vi "ziExample-Scope.vi"() -> ()   [LabVIEW 2009]
doc: "Control a Zurich instrument device via the LabOne Labview API. \nRequirements: Zurich Instruments MFLI, HF2 or UHFLI \nThis example retrieves scope data from a Zurich Instruments instrument.\n\n© Zurich Instruments AG, www.zhinst.com"
uses:
  <instrlib>/Zurich Instruments LabOne/Public/Configure/ziSetValueDouble.vi
  <instrlib>/Zurich Instruments LabOne/Public/Configure/ziGetValueString.vi
  <instrlib>/Zurich Instruments LabOne/Public/Configure/ziSetValueDoubleArray.vi
  <instrlib>/Zurich Instruments LabOne/Public/Configure/ziGetValueDouble.vi
  <instrlib>/Zurich Instruments LabOne/Public/Data/ziGetEventScopeWaveEX.vi
  <instrlib>/Zurich Instruments LabOne/Zurich Instruments LabOne.lvlib
  <vilib>/Analysis/NI_AALPro.lvlib
panel:
  out "ScopeWave Out":T1(array[cluster])
  out "Error Out":errorcluster
  in  "Address":string="DEV"
  out "FFT":T2(graph)
  out "Selected Device":string
  out "Waveform":cluster{"dt (?)":dbl, "dt (s)":dbl, dbl[]}[](graph)
  in  "stop":bool
  # "ziExample-Scope.vi:\nThis example is legacy and please use ziExample-Module-Scope.vi"
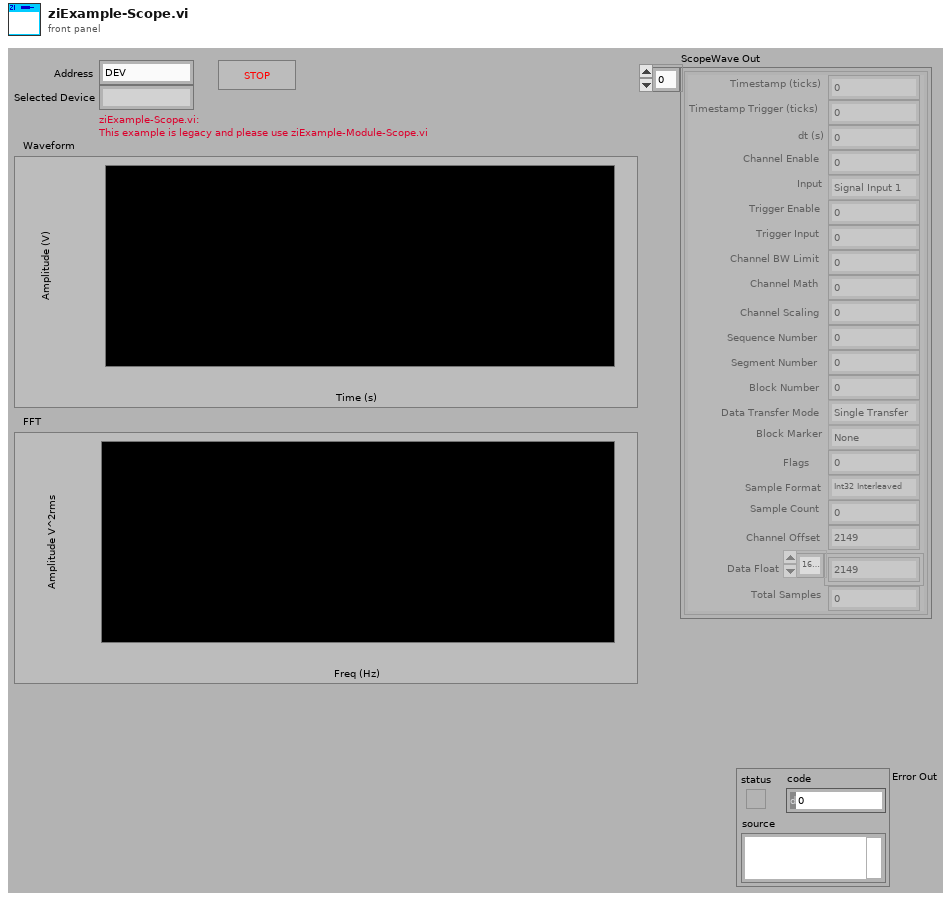
[diagram p1: front panel]
types:
  T1 = cluster{"Timestamp (ticks)":u64, "Timestamp Trigger (ticks)":u64, "dt (s)":dbl, "Channel Enable":u8, "Input":enum8{"Signal Input 1", "Signal Input 2", "Trigger Input 1", "Trigger Input 2", "Aux Output 1", "Aux Output 2", "Aux Output 3", "Aux Output 4", "Aux Input 1", "Aux Input 2"}, "Trigger Enable":u64, "Trigger Input":u64, "Channel BW Limit":u8, "Channel Math":u8, "Channel Scaling":sgl, "Sequence Number":u32, "Segment Number":u32, "Block Number":u32, "Data Transfer Mode":enum8{"Single Transfer", "Block Transfer", "Continuous Transfer", "FFT Single Transfer"}, "Block Marker":enum8{"None", "End of Block"}, "Flags":u8, "Sample Format":enum8{"Int16", "Int32", "Float32", "reserved", "Int16 Interleaved", "Int32 Interleaved", "Float32 Interleaved"}, "Sample Count":u32, "Channel Offset":dbl, "Data Float":sgl[], "Total Samples":u64}[]
  T2 = cluster{"dt (?)":dbl, "df":dbl, "Power Spectrum (V^2 rms)":dbl[]}[]
  T3 = typedef "Zurich Instruments LabOne.lvlib/ziTypeHandle.ctl" = cluster{"handleValid":bool, "Conn":u64, "Path Prefix":string, "Handle":u64, "Connected":bool, "Clockbase(s)":dbl}
  T4 = typedef "Zurich Instruments LabOne.lvlib/ziTypePollType.ctl" = enum16{"NONE", "DOUBLE_DATA", "INTEGER_DATA", "DEMOD_SAMPLE", "SCOPE_WAVE_HF2", "AUXIN_SAMPLE", "DIO_SAMPLE", "BYTE_ARRAY", "PWA_WAVE", "9", "10", "11", "12", "13", "14", "15", "TREE_CHANGE_DEPRI", "17", "ERROR", "19", "20", "21", "22", "23", "24", "25", "26", "27", "28", "29", "30", "31", "DOUBLE_DATA_TS", "INTEGER_DATA_TS", "34", "SCOPE_WAVE", "SCOPE_WAVE_EX", "37", "BYTE_ARRAY_TS", "39", "40", "41", "42", "43", "44", "45", "CNT_DATA", "47", "TREE_CHANGE", "49", "50", "51", "52", "53", "54", "55", "56", "57", "58", "59", "60", "61", "62", "63", "SWEEPER_DATA", "SPECTRUM_DATA", "ADVISOR_DATA", "VECTOR_DATA", "IMP_DATA"}
  T5 = cluster{"dt (?)":dbl, "df":dbl, "Power Spectrum (V^2 rms)":dbl[]}
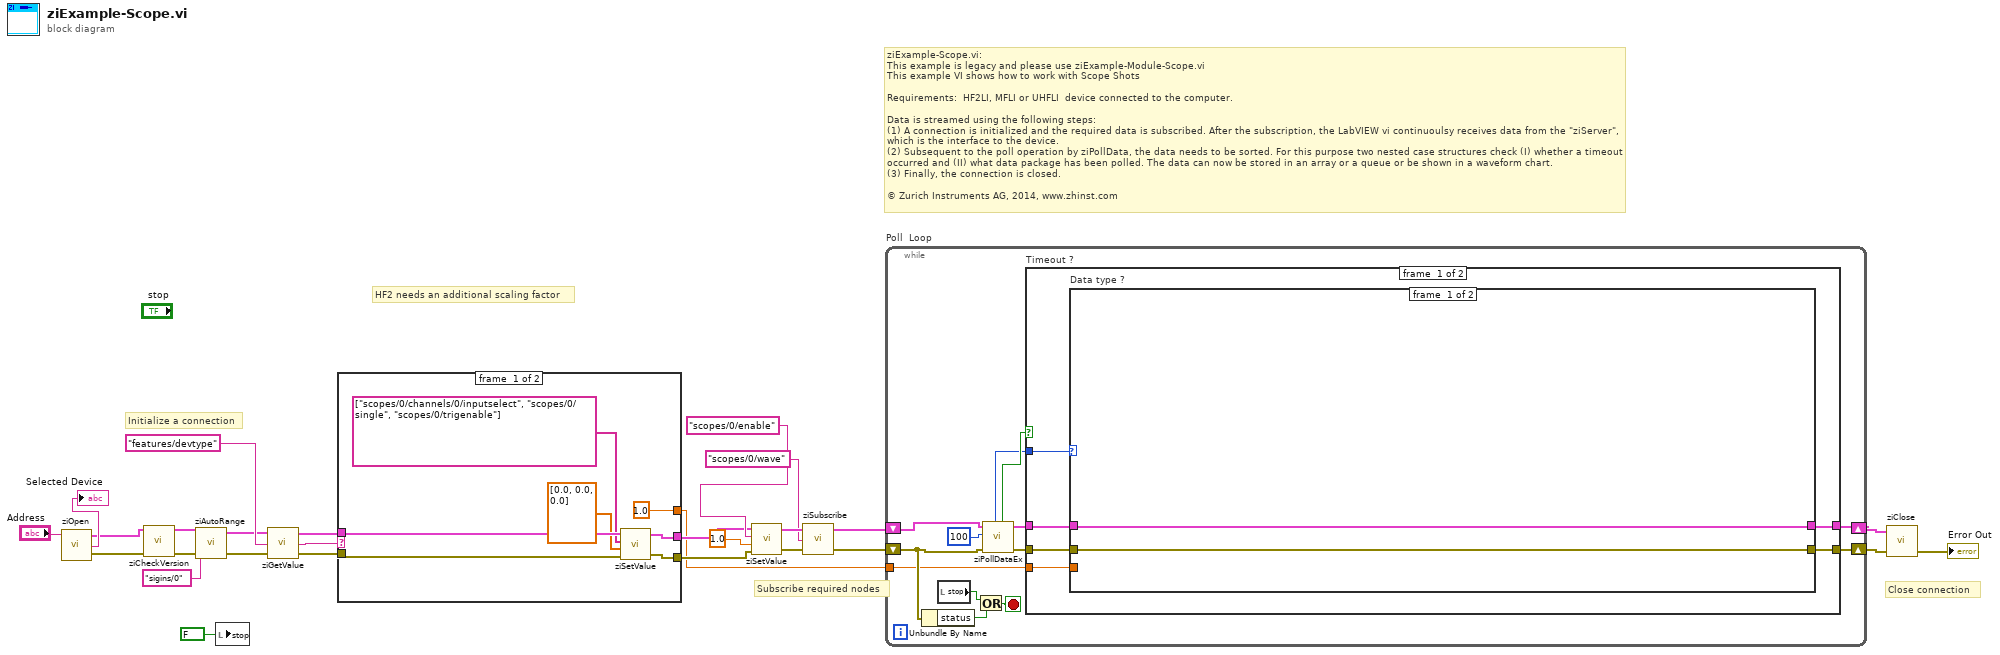
[diagram p0: block diagram]
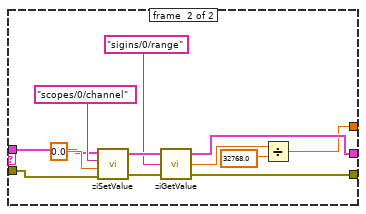
[diagram p2: hidden frame]
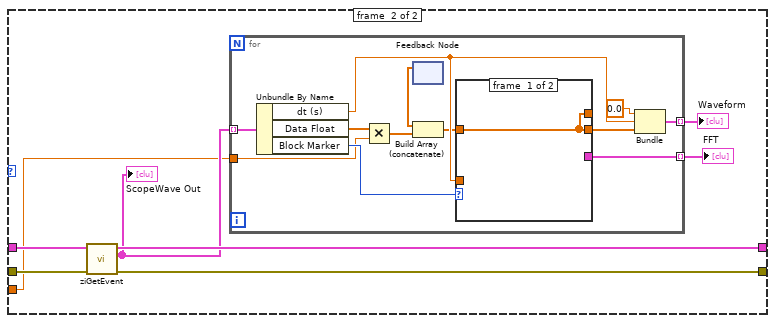
[diagram p3: hidden frame]
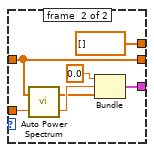
[diagram p4: hidden frame]
diagram:
  # "Close connection"
  # "HF2 needs an additional scaling factor"
  # "Initialize a connection"
  # "Subscribe required nodes"
  # "ziExample-Scope.vi:\nThis example is legacy and please use ziExample-Module-Scope.vi\nThis example VI shows how to work with Scope Shots\n\nRequirements:  HF2LI, MFLI or UHFLI  device connected to the computer.\n\nData is streamed using the following steps:\n(1) A connection is initialized and the required data is subscribed. After the subscription, the LabVIEW vi continuoulsy receives data from the \"ziServer\", which is the interface to the device. \n(2) Subsequent to the poll operation by ziPollData, the data needs to be sorted. For this purpose two nested case structures check (I) whether a timeout occurred and (II) what data package has been polled. The data can now be stored in an array or a queue or be shown in a waveform chart. \n(3) Finally, the connection is closed. \n\n© Zurich Instruments AG, 2014, www.zhinst.com"
  n1 = call <instrlib>:"ziOpen.vi"("Address"="Address") -> ("Error Out"=w2:errorcluster, "Selected Device"=→"Selected Device":string, "HandleOut"=w1:T3)  [unwired: 1 in, 2 out]
  n2 = call <instrlib>:"ziCheckVersion.vi"("Handle In"=w1, "Error In"=w2) -> ("Handle Out"=w4:T3, "Error Out"=w3:errorcluster)  [unwired: 11 in, 1 out]
  n3 = call <instrlib>:"ziAutoRange.vi"("Error in"=w3, "Path"="sigins/0", "Handle in"=w4) -> ("Error out"=w6:errorcluster, "Handle out"=w7:T3)  [unwired: 6 in, 1 out]
  n4 = local write "stop"(FALSE ("Record")) -> ()
  n5 = call-poly <instrlib>:"ziGetValue.vi"("error in"=w6, "Path"="features/devtype", "Handle In"=w7) -> ("error out"=w14:errorcluster, "Value"=w12:string, "Handle Out"=w13:T3)
  n6 = case shown="Default" w12 {
    tunnel: w13 -> [w34 w44]
    tunnel: w14 -> [w33 w43]
    tunnel: [w32 w40] -> w16
    tunnel: [w31 w41] -> w15
    tunnel: [1.0 w36] -> w10
    frame #0 {
      n7 = call-poly <instrlib>:"ziSetValue.vi"("Error In"=w33, "Values"=dbl[] [0.0, 0.0, 0.0], "Paths"=string[] ["scopes/0/channels/0/inputselect", "scopes/0/single", "scopes/0/trigenable"], "Handle In"=w34) -> ("Error Out"=w32:errorcluster, "Handle Out"=w31:T3)  [unwired: 1 in]
    }
    frame #1 {
      n8 = call-poly <instrlib>:"ziSetValue.vi"("Error In"=w43, "Value"=0.0, "Path"="scopes/0/channel", "Handle In"=w44) -> ("Error Out"=w39:errorcluster, "Handle Out"=w42:T3)  [unwired: 1 in]
      n9 = call-poly <instrlib>:"ziGetValue.vi"("error in"=w39, "Path"="sigins/0/range", "Handle in"=w42) -> ("error out"=w40:errorcluster, "Value"=w37:dbl, "Handle out"=w41:T3)
      n10 = Divide(x=w37, y=32768.0) -> (x/y=w36:dbl)
    }
  }
  n11 = call-poly <instrlib>:"ziSetValue.vi"("Error In"=w16, "Value"=1.0, "Path"="scopes/0/enable", "Handle In"=w15) -> ("Error Out"=w20:errorcluster, "Handle Out"=w21:T3)  [unwired: 1 in]
  n12 = call <instrlib>:"ziSubscribe.vi"("error in"=w20, "Path ()"="scopes/0/wave" ("path"), "Handle In"=w21) -> ("error out"=w24:errorcluster, "Handle Out"=w8:T3)  [unwired: 1 in]
  n13 = while "Poll  Loop" {
    shift-right: [w55] -> w25
    shift-left: w8 -> [w59]
    shift-right: [w53] -> w26
    shift-left: w24 -> [w52]
    tunnel: w10 -> [w48]
    stop <- w49 stop-if-true
    n14 = Unbundle By Name(w52) -> ("status"=w51:bool)
    n15 = local read "stop"() -> (w50:bool)
    n16 = Or(x=w50, y=w51) -> (x .or. y?=w49:bool)
    n17 = call <instrlib>:"ziPollDataEx.vi"("error in"=w52, "Timeout ms (50)"=100 ("TimeOut ms (50)"), "Handle In"=w59) -> ("error out"=w54:errorcluster, "Handle Out"=w56:T3, "Timed Out"=w57:bool, "ziValueType"=w47:T4)  [unwired: 1 in, 4 out]
    n18 = case "Timeout ?" shown="False" w57 {
      tunnel: w56 -> [w65 w98]
      tunnel: [w64 w98] -> w55
      tunnel: w54 -> [w63 w97]
      tunnel: [w62 w97] -> w53
      tunnel: w48 -> [w61 _]
      tunnel: w47 -> [w60 _]
      frame #0 {
        n19 = case "Data type ?" shown="\"SCOPE_WAVE\"" w60 {
          tunnel: w65 -> [w67 w75]
          tunnel: [w67 w74] -> w64
          tunnel: w63 -> [w66 w73]
          tunnel: [w66 w72] -> w62
          tunnel: w61 -> [_ w69]
          frame #0 {
          }
          frame #1 {
            n20 = call-poly <instrlib>:"ziGetEvent.vi"("Error In"=w73, "Handle In"=w75) -> ("Error Out"=w72:errorcluster, "ScopeWave Out"=w71:T1, "Handle Out"=w74:T3)  [unwired: 7 in]
            "ScopeWave Out" <- w71
            n21 = for {
              tunnel: w71 -> [w88] mode=indexing
              tunnel: [w86] -> w70 mode=indexing
              tunnel: [w85] -> w68 mode=indexing
              tunnel: w69 -> [w82]
              n22 = Unbundle By Name(w88) -> ("dt (s)"=w84:dbl, "Data Float"=w81:sgl[], "Block Marker"=w83:enum8{"None", "End of Block"})
              n23 = Multiply(x=w81, y=w82) -> (x*y=w78:dbl[])
              n24 = feedback #1() -> (w80:dbl[])  [unwired: 1 in]
              n25 = Build Array (concatenate)(w80, w78) -> (w79:dbl[])
              n26 = case shown="\"End of Block\"" w83 {
                tunnel: [_ w94] -> w85
                tunnel: w84 -> [_ w93]
                tunnel: w79 -> [w89 w91]
                tunnel: [w89 dbl[] []] -> w77
                tunnel: [w89 w91] -> w76
                frame #0 {
                }
                frame #1 {
                  n27 = call <vilib>:"Auto Power Spectrum.vi"("dt"=w93, "Signal (V)"=w91) -> ("df"=w95:dbl, "Power Spectrum (V^2 rms)"=w90:dbl[])
                  n28 = Bundle("dt (?)"=0.0, "df"=w95, "Power Spectrum (V^2 rms)"=w90) -> (w94:T5)  [unwired: 1 in]
                }
              }
              n29 = Bundle("dt (?)"=0.0, "dt (s)"=w84, w76) -> (w86:cluster{"dt (?)":dbl, "dt (s)":dbl, dbl[]})  [unwired: 1 in]
            }
            "Waveform" <- w70
            "FFT" <- w68
          }
        }
      }
      frame #1 {
        # "Timeout, no action."
      }
    }
  }
  n30 = call <instrlib>:"ziClose.vi"("Error In"=w26, "Handle In"=w25) -> ("Error Out"=→"Error Out":errorcluster)  [unwired: 3 out]
